vi "PH_Watchdog.set i Attr.vi"(2 "error in (no error)":errorcluster) -> (0 "error out":errorcluster, 1 "i attribute":T1 {"All"."Status" items=["no info", "off/false/out", "on/true/in", "Failure", "Alarm", "Status 1", "Status 2", "Status 3"]})   [LabVIEW 2014, in "PH_Watchdog.lvlib"]
uses:
  PH_Watchdog.lvlib
  PH_Watchdog.i attribute.ctl
  PH_Watchdog.Dataset.ctl
  PH_Basics/PH_StatusHandler/PH_StatusHandler.Status.ctl
  PH_Basics/PH_Common/PH_Common.lvlib
  PH_Basics/PH_StatusHandler/PH_StatusHandler.lvlib
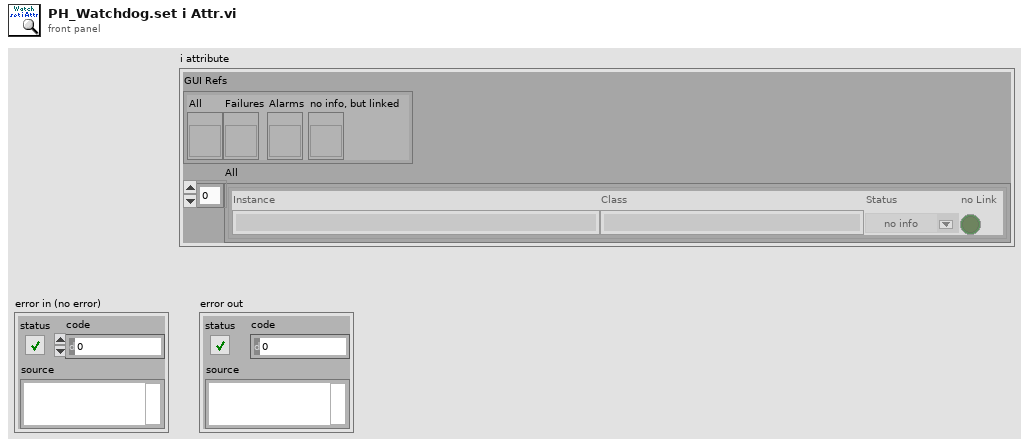
[diagram p1: front panel]
types:
  T1 = typedef "PH_Watchdog.lvlib/PH_Watchdog.i attribute.ctl" = cluster{"GUI Refs":cluster{"All":refnum<vi>, "Failures":refnum<vi>, "Alarms":refnum<vi>, "no info, but linked":refnum<vi>}, "All":T2[]}
  T2 = typedef "PH_Watchdog.lvlib/PH_Watchdog.Dataset.ctl" = cluster{"Instance":string, "Class":string, "Status":T3, "no Link":bool}
  T3 = typedef "PH_StatusHandler.lvlib/PH_StatusHandler.Status.ctl" = i16
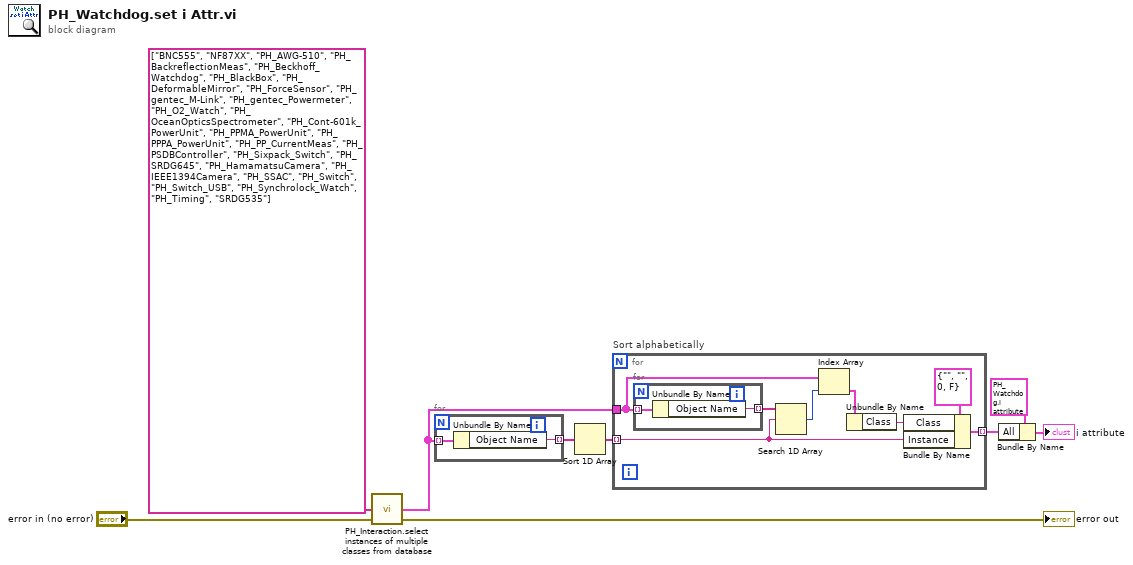
[diagram p0: block diagram]
diagram:
  n1 = call "PH_Interaction.select instances of multiple classes from database.vi"("error in (no error)"="error in (no error)", "Classes Input"=string[] ["BNC555", "NF87XX", "PH_AWG-510", "PH_BackreflectionMeas", "PH_Beckhoff_Watchdog", "PH_BlackBox", "PH_DeformableMirror", "PH_ForceSensor", "PH_gentec_M-Link", "PH_gentec_Powermeter", "PH_O2_Watch", "PH_OceanOpticsSpectrometer", "PH_Cont-601k_PowerUnit", "PH_PPMA_PowerUnit", "PH_PPPA_PowerUnit", "PH_PP_CurrentMeas", "PH_PSDBController", "PH_Sixpack_Switch", "PH_SRDG645", "PH_HamamatsuCamera", "PH_IEEE1394Camera", "PH_SSAC", "PH_Switch", "PH_Switch_USB", "PH_Synchrolock_Watch", "PH_Timing", "SRDG535"]) -> ("error out"=→"error out":errorcluster, "Query Result"=w1:cluster{"Object Name":string, "Class":string}[])  [unwired: 2 in]
  n2 = for {
    tunnel: w1 -> [w11] mode=indexing
    tunnel: [w10] -> w6 mode=indexing
    n3 = Unbundle By Name(w11) -> ("Object Name"=w10:string)
  }
  n4 = Sort 1D Array(array=w6) -> (sorted array=w2:string[])
  n5 = for "Sort alphabetically" {
    tunnel: [w18] -> w3 mode=indexing
    tunnel: w2 -> [w16] mode=indexing
    tunnel: w1 -> [w14]
    n6 = for {
      tunnel: w14 -> [w21] mode=indexing
      tunnel: [w20] -> w17 mode=indexing
      n7 = Unbundle By Name(w21) -> ("Object Name"=w20:string)
    }
    n8 = Search 1D Array(1D array=w17, element=w16) -> (index of element=w15:i32)  [unwired: 1 in]
    n9 = Index Array(array=w14, index=w15) -> (element=w13:cluster{"Object Name":string, "Class":string})
    n10 = Unbundle By Name(w13) -> ("Class"=w12:string)
    n11 = Bundle By Name(cluster=T2 {"Instance"="", "Class"="", "Status"=0, "no Link"=FALSE} ("Dataset"), "Class"=w12, "Instance"=w16) -> (w18:T2)
  }
  n12 = Bundle By Name(cluster=T1 {"GUI Refs"={"All"=refnum, "Failures"=refnum, "Alarms"=refnum, "no info, but linked"=refnum}, "All"=[]} ("i attribute"), "All"=w3) -> (→"i attribute":T1)
